vi "frontend2.vi"() -> ()   [LabVIEW 2011]
uses:
  custom_modules/typedefs/preset_control_cluster.ctl
  custom_modules/typedefs/control_cluster.ctl
  custom_modules/typedefs/origin_controls.ctl
  custom_modules/typedefs/single_step_controls.ctl
  custom_modules/typedefs/camera_settings_new.ctl
  custom_modules/typedefs/states_v2.ctl
  <vilib>/event_ctls.llb/eventvkey.ctl
  custom_modules/typedefs/dynamic_data.ctl
  <vilib>/vision/Image Controls.llb/IMAQ Image.ctl
  custom_modules/typedefs/image_type.ctl
  <vilib>/Utility/error.llb/DialogType.ctl
  stage_modules/Globals.vi
  <userlib>/qcam/QCam.llb/QCam Grab Abort.vi
  <vilib>/vision/NI_Vision_Development_Module.lvlib
panel:
  in  "test start time":u32
  out "abort test":bool
  out "error display":errorcluster
  in  "Tab Control":enum32{"Settings", "Advanced"}(tab)
  in  "Preset controls":T1 {"Presets" items=["500sep.preset", "test1.preset", "test2.preset", "test3.preset"]}
  in  "Movement controls":T2={"Nx"=10, "Ny"=10, "X separation"=100, "Y separation"=100}
  in  "File name base":string="<title>_<length>_<sampleID>_<stain>"
  in  "Run test button":bool
  in  "close button":bool
  in  "Origin controls":T3
  in  "Single step controls":T4
  in  "Camera settings":T5={"Gain"=1.0, "Exposure (s)"=0.05, "Preview binning"=2, "Capture binning"=0, "auto expose button"=FALSE} {"Capture binning" items=["1x1", "2x2", "4x4", "8x8"]; "Preview binning" items=["1x1", "2x2", "4x4", "8x8"]; "Exposure (s)" scale=1e-05..1000.0 scale format="%^#_1e"; "Gain" scale=0.451..21.5 scale format="%#_3g"}
  out "Histogram":T6(graph)
  out "Preview":T7(plugin-control)
  in  "camera button":bool
  in  "Image Output directory":path=path "C:/Users/0800706m/Documents/output"
  out "connection indicator":bool
  out "Scan map viewer":T7(plugin-control)
  out "elapsed time":string
  out "estimated remaining":string
  in  "Well numbering mode":u16(ring)=1 items=["X and Y numbers", "Numbers and letters"]
  in  "No. of wells Y":i32=1
  in  "No. of wells X":i32=1
  in  "Well separation Y":dbl=899.0
  in  "Well separation X":dbl=899.0
  in  "PC connection port":u16(ring)=3 items=["PCI board", "COM 1", "TPL1", "COM3"]
  in  "No. of images in focal stack":i32=1
  in  "Focal stack separation":dbl=1.0
  in  "Preset directory":path=path "C:/Users/0800706m/Documents/microscope_software/presets"
  in  "Additional delay between captures (ms)":dbl=1000.0
  in  "emergency stop":bool
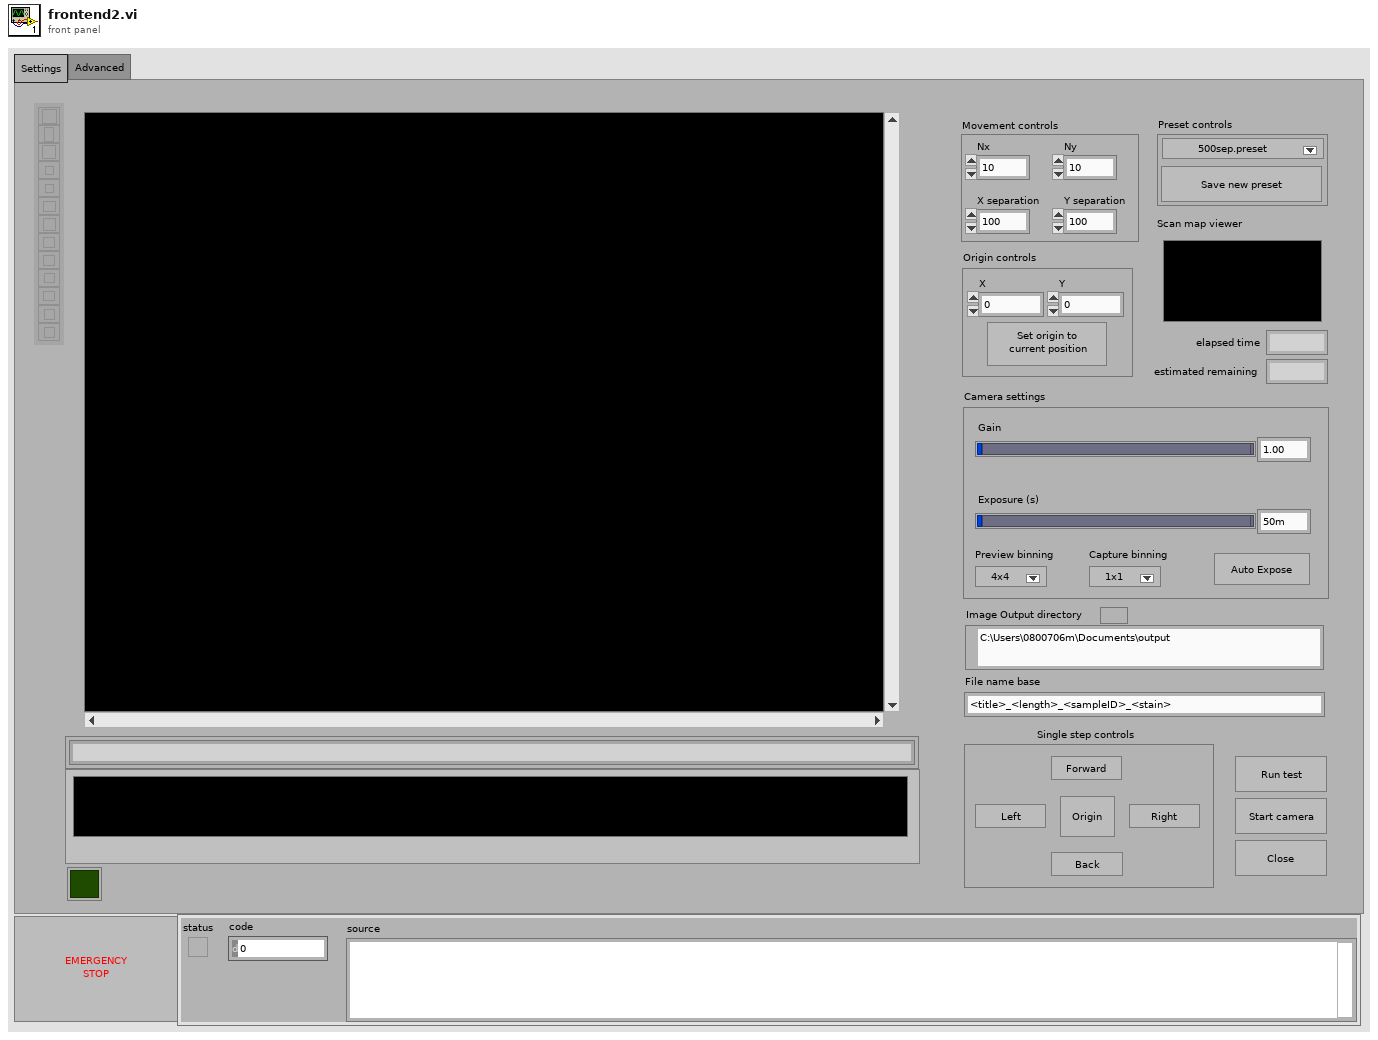
[diagram p1: front panel]
types:
  T1 = typedef "preset_control_cluster.ctl" = cluster{"Presets":u16, "save preset button":bool}
  T2 = typedef "control_cluster.ctl" = cluster{"Nx":i32, "Ny":i32, "X separation":i32, "Y separation":i32}
  T3 = typedef "origin_controls.ctl" = cluster{"X":dbl, "Y":dbl, "set origin button":bool}
  T4 = typedef "single_step_controls.ctl" = cluster{"move to origin button":bool, "Left":bool, "Right":bool, "Back":bool, "Forward":bool}
  T5 = typedef "camera_settings_new.ctl" = cluster{"Gain":dbl, "Exposure (s)":dbl, "Preview binning":u16, "Capture binning":u16, "auto expose button":bool}
  T6 = cluster{"Starting Value":sgl, "Incremental Value":sgl, "Histogram":u32[]}
  T7 = typedef "IMAQ Image.ctl" = refnum<image>
  T8 = typedef "states_v2.ctl" = enum16{"Init", "Preview", "Test init", "Test run", "Test clean", "Close"}
  T9 = typedef "dynamic_data.ctl" = cluster{"PRIORLib.IScanOut":refnum<k7>, "PRIORLib.IStageOut":refnum<k7>, "PRIORLib.IFilterOut":refnum<k7>, "PRIORLib.IZOut":refnum<k7>, "cameraID":u32, "Image Out":T7, "focal map fileref":refnum<file>, "Scan map":T7, "start time":u32}
  T10 = enum8{"Enabled", "Disabled", "Disabled and Grayed Out"}
  T11 = typedef "image_type.ctl" = enum16{"preview_image", "capture_image"}
  T12 = enum32{"gain", "offset", "exposure", "binning", "horizontal binning", "vertical binning", "readout speed", "trigger type", "lcd filter", "cooler", "exposure red", "exposure blue", "image format", "roi x", "roi y", "roi width", "roi height", "reserved1", "shutter state", "reserved2", "sync-b out", "reserved3", "intensifier gain", "trigger delay", "camera mode", "normalized gain", "normalized intenifier gain DB", "doPostProcessing", "postProcessGainRed", "postProcessGainGreen", "postProcessGainBlue", "postProcessBayerAlgorithm", "postProcessImageFormat", "fan", "blackout mode", "high sensitivity", "Readout Port", "EM Gain", "open delay", "close delay", "clearing mode"}
  T13 = enum16{"open", "replace", "create", "open or create", "replace or create", "replace or create with confirmation"}
  T14 = typedef "Image Type" = u32
  T15 = cluster{"Value":bool, "Value":bool, "Value":bool, "Value":bool, "Value":bool}
  T16 = cluster{"Global Rectangle":i32[], "Contours":cluster{"Contour Type":u32, "ROI Type":u32, "Points":i32[]}[]}
  T17 = typedef "DialogType.ctl" = u16
  T18 = cluster{"stage adjusted":bool, "stage adjusted":bool, "stage adjusted":bool, "stage adjusted":bool, "stage adjusted":bool}
  T19 = cluster{"Focus position":dbl, "Number of captures":i32}
  T20 = typedef "eventvkey.ctl" = enum16{"ASCII", "Enter", "Return", "Shift", "Ctrl", "Alt", "Cmd", "Opt", "Caps", "NumLock", "Clear", "Break", "Up", "Down", "Left", "Right", "Insert", "Delete", "Home", "End", "PageUp", "PageDown", "Escape", "Help", "Pause", "ScrollLock", "F1", "F2", "F3", "F4", "F5", "F6", "F7", "F8", "F9", "F10", "F11", "F12", "F13", "F14", "F15", "F16", "F17", "F18", "F19", "F20", "F21", "F22", "F23", "F24", "Play", "VolumeUp", "VolumeDown", "Mute", "Two Byte Char"}
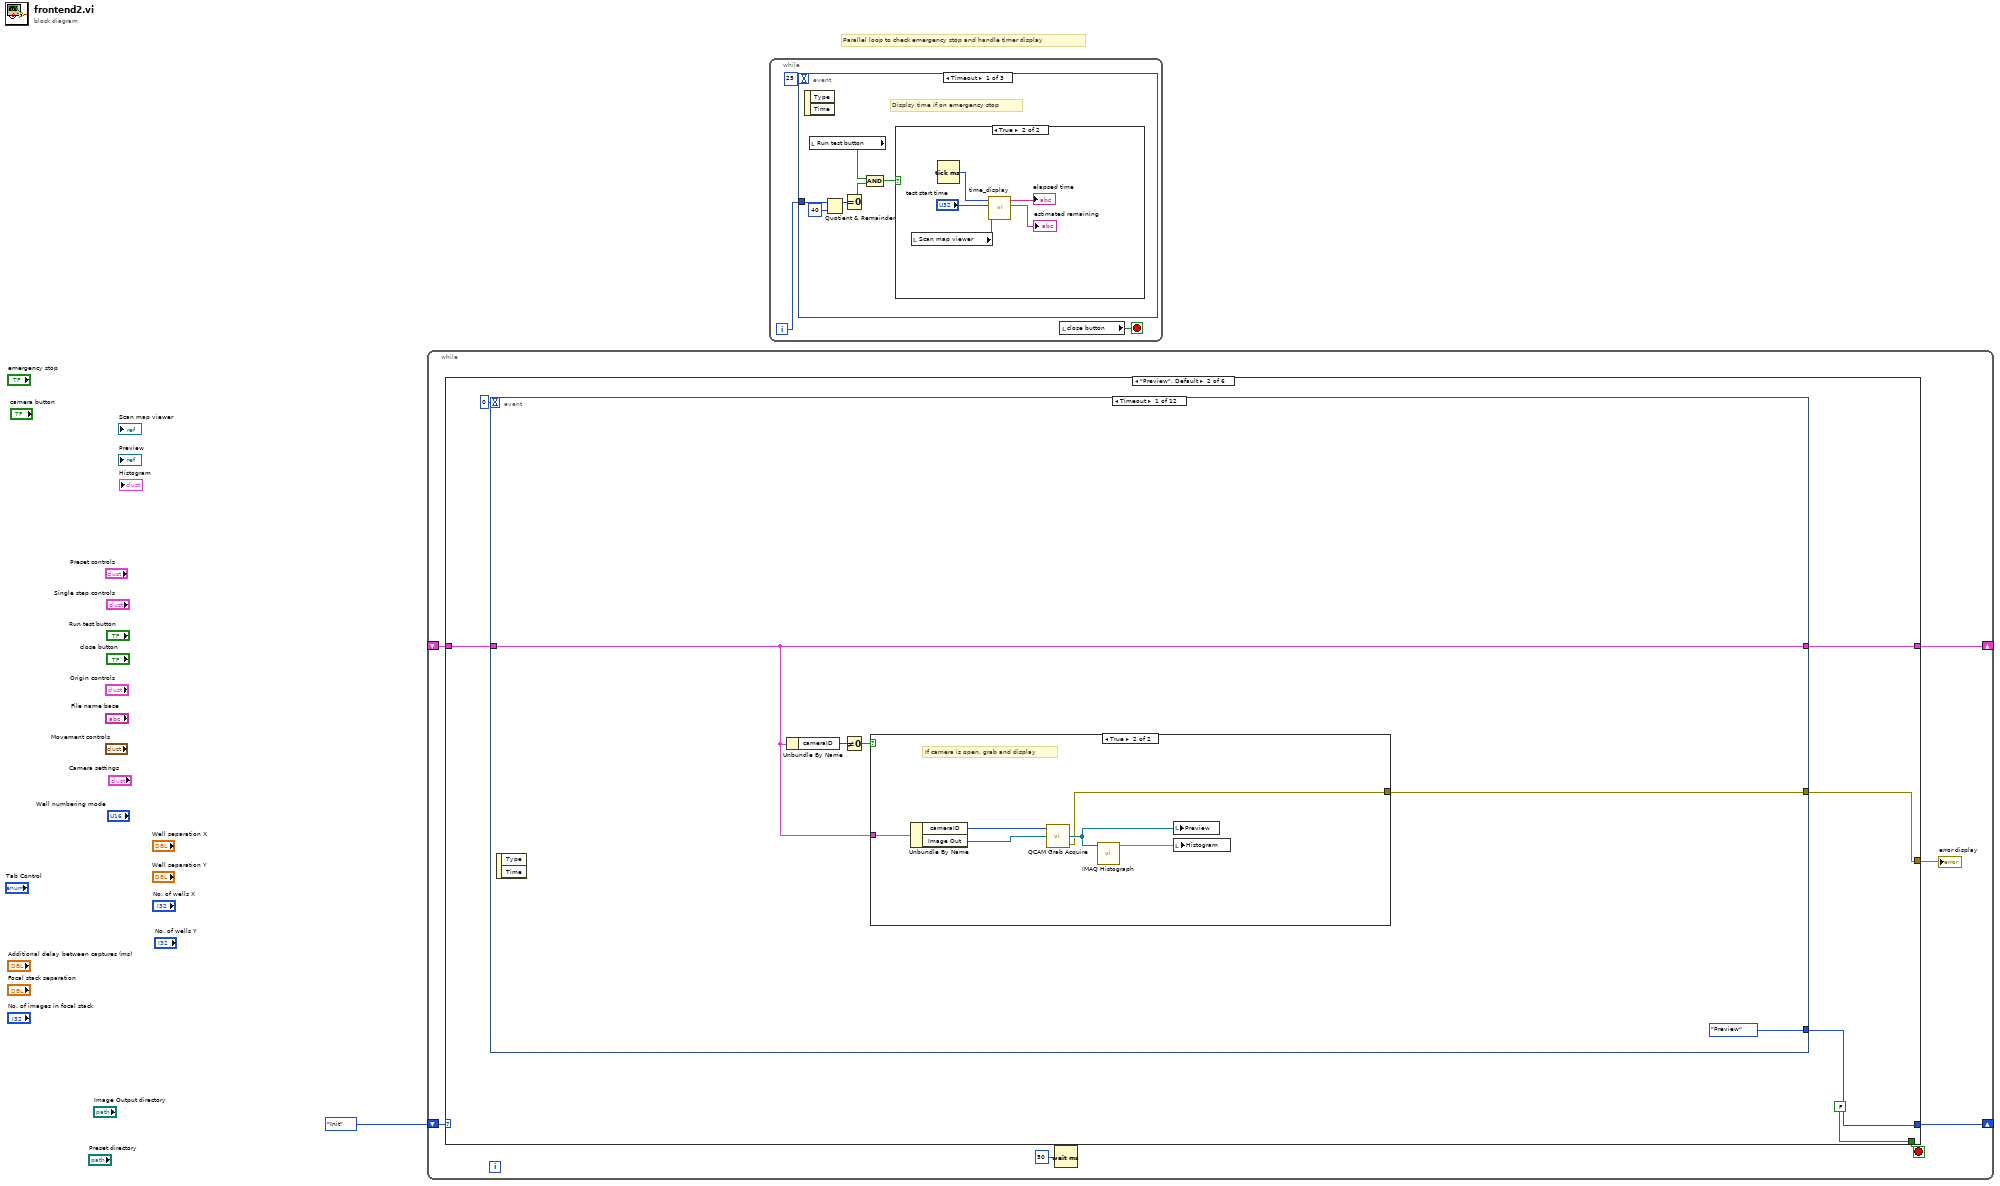
[diagram p0: block diagram]
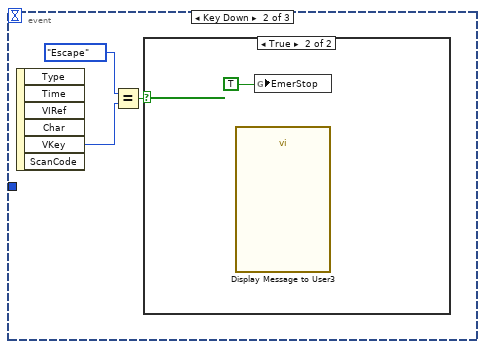
[diagram p3: hidden frame]
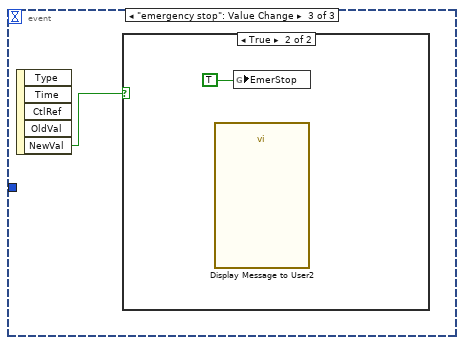
[diagram p5: hidden frame]
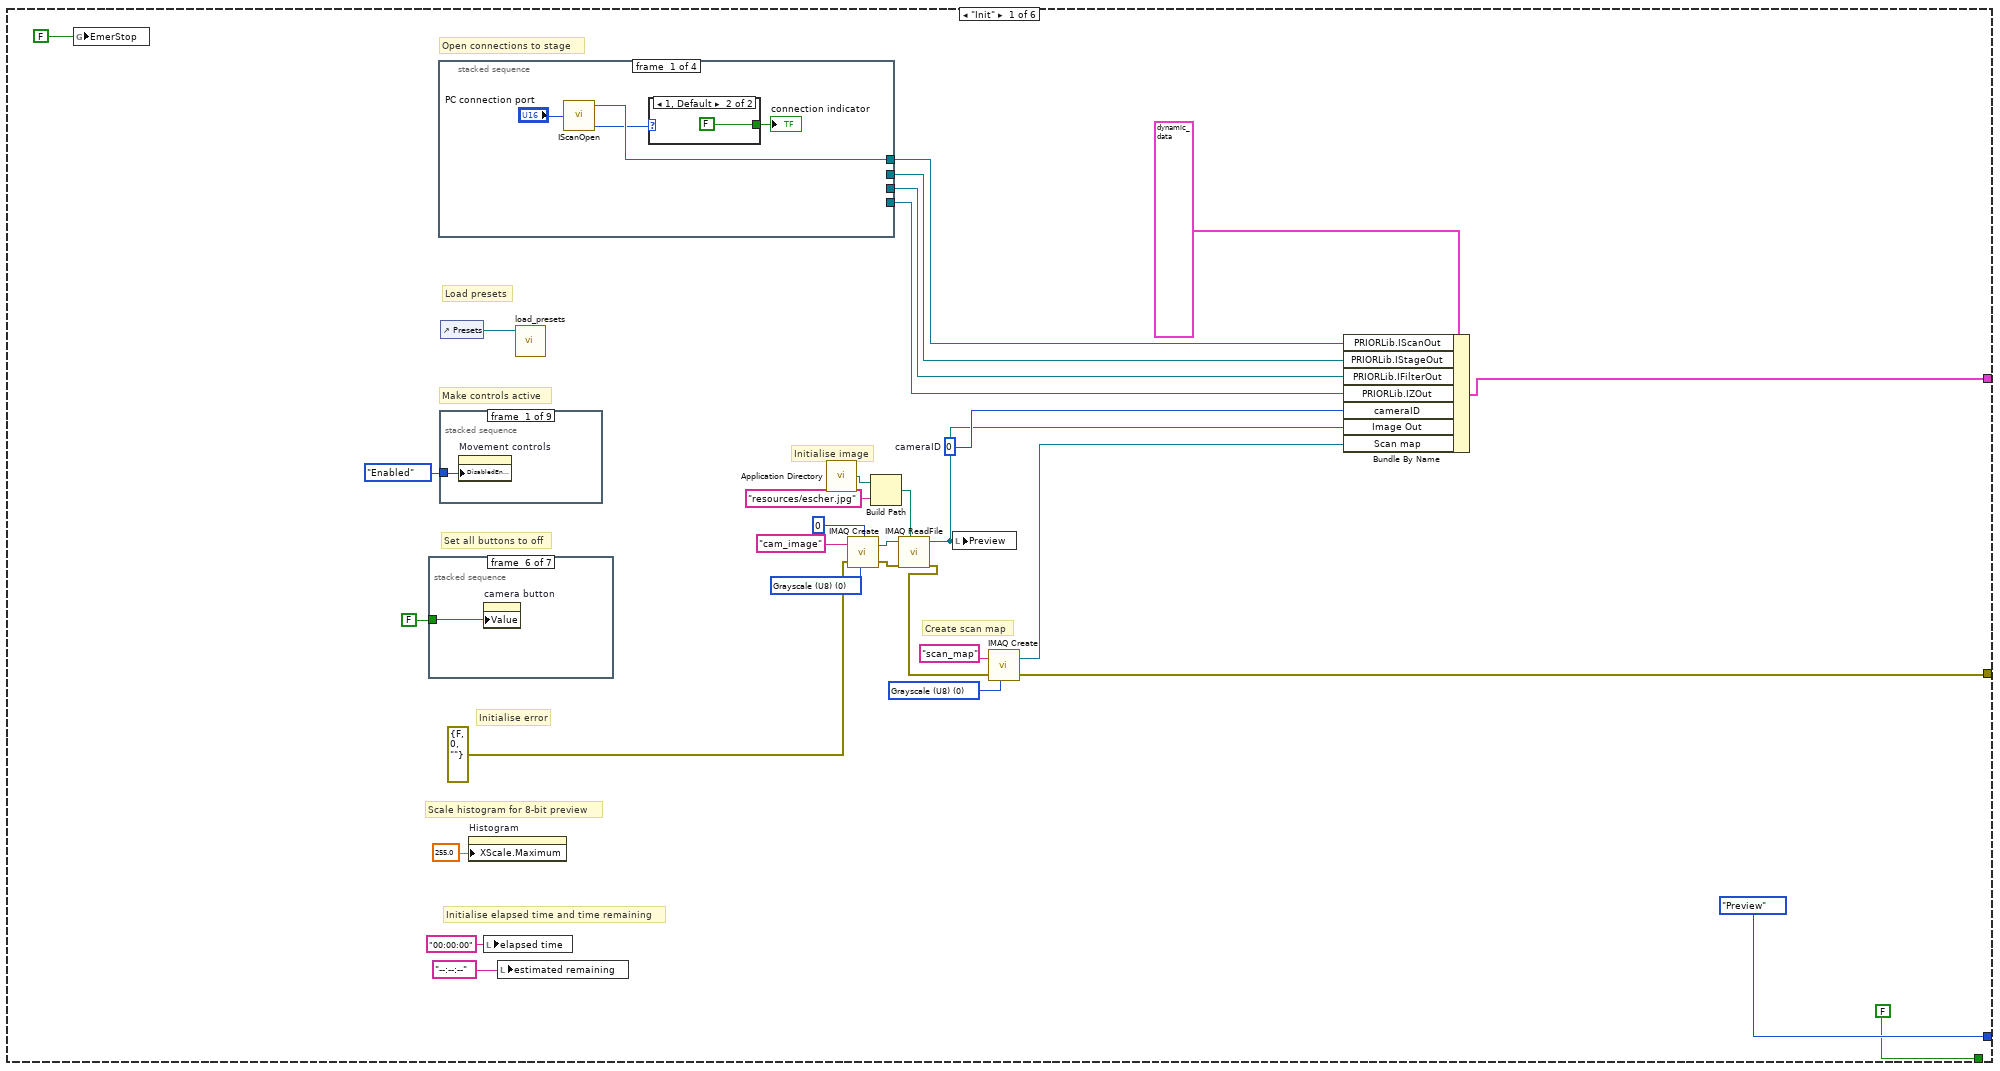
[diagram p7: hidden frame]
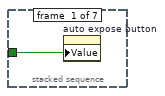
[diagram p8: hidden frame]
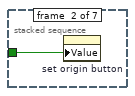
[diagram p9: hidden frame]
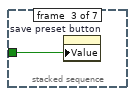
[diagram p10: hidden frame]
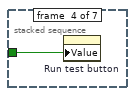
[diagram p11: hidden frame]
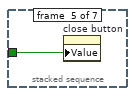
[diagram p12: hidden frame]
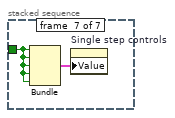
[diagram p13: hidden frame]
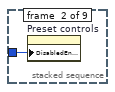
[diagram p14: hidden frame]
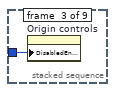
[diagram p15: hidden frame]
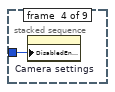
[diagram p16: hidden frame]
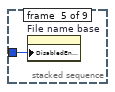
[diagram p17: hidden frame]
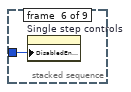
[diagram p18: hidden frame]
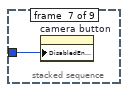
[diagram p19: hidden frame]
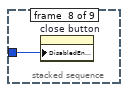
[diagram p20: hidden frame]
diagram:
  # "Parallel loop to check emergency stop and handle timer display"
  n1 = while {
    shift-right: [w7] -> _
    shift-left: states_v2."Init" -> [w8]
    shift-right: [w5] -> _
    shift-left: _ -> [w2]
    stop <- w6 stop-if-true
    n2 = case shown="\"Preview\", Default" w8 {
      tunnel: [states_v2."Preview" w72 w315 states_v2."Test clean" states_v2."Preview" states_v2."Close"] -> w7
      tunnel: [FALSE FALSE FALSE FALSE FALSE TRUE] -> w6
      tunnel: [w19 w70 w280 w341 w542 T9 {"PRIORLib.IScanOut"=refnum, "PRIORLib.IStageOut"=refnum, "PRIORLib.IFilterOut"=refnum, "PRIORLib.IZOut"=refnum, "cameraID"=0, "Image Out"=refnum, "focal map fileref"=refnum, "Scan map"=refnum, "start time"=0}] -> w5
      tunnel: w2 -> [_ w69 w281 w341 w534 w558]
      tunnel: [w13 w68 w279 _ w531 w556] -> w3
      frame "Init" {
        w17 = T14 0 items=["Grayscale (U8)", "Grayscale (I16)", "Grayscale (SGL)", "Complex (CSG)", "RGB (U32)", "HSL (U32)", "RGB (U64)", "Grayscale (U16)"] ("Image Type")
        w29 = T14 0 items=["Grayscale (U8)", "Grayscale (I16)", "Grayscale (SGL)", "Complex (CSG)", "RGB (U32)", "HSL (U32)", "RGB (U64)", "Grayscale (U16)"] ("Image Type")
        w28 = u32 0  # cameraID
        # "Initialise elapsed time and time remaining"
        # "Create scan map"
        # "Initialise image"
        # "Scale histogram for 8-bit preview"
        # "Initialise error"
        # "Set all buttons to off"
        # "Make controls active"
        # "Open connections to stage"
        # "Load presets"
        n3 = global write "Globals.vi" "EmerStop"(FALSE) -> ()
        n4 = stacked-sequence {
          tunnel: FALSE ("Value") -> [w40 w41 w42 w43 w44 w45 w46]
          frame #0 {
            n5 = property on="auto expose button" class="Bool (strict)"("Value"=w40) -> ()  [unwired: 2 in, 2 out]
          }
          frame #1 {
            n6 = property on="set origin button" class="Bool (strict)"("Value"=w41) -> ()  [unwired: 2 in, 2 out]
          }
          frame #2 {
            n7 = property on="save preset button" class="Bool (strict)"("Value"=w42) -> ()  [unwired: 2 in, 2 out]
          }
          frame #3 {
            n8 = property on="Run test button" class="Bool (strict)"("Value"=w43) -> ()  [unwired: 2 in, 2 out]
          }
          frame #4 {
            n9 = property on="close button" class="Bool (strict)"("Value"=w44) -> ()  [unwired: 2 in, 2 out]
          }
          frame #5 {
            n10 = property on="camera button" class="Bool (strict)"("Value"=w45) -> ()  [unwired: 2 in, 2 out]
          }
          frame #6 {
            n11 = Bundle("Value"=w46, "Value"=w46, "Value"=w46, "Value"=w46, "Value"=w46) -> (w47:T15)  [unwired: 1 in]
            n12 = property on="Single step controls" class="Clust (strict)"("Value"=w47) -> ()  [unwired: 2 in, 2 out]
          }
        }
        n13 = stacked-sequence {
          tunnel: [w60 _ _ _] -> w10
          tunnel: [_ w63 _ _] -> w35
          tunnel: [_ _ w64 _] -> w34
          tunnel: [_ _ _ w65] -> w33
          frame #0 {
            n14 = call "IScanOpen.vi"("Port"="PC connection port") -> ("PRIORLib.IScanOut"=w60:refnum<k7>, "Return"=w59:i32)  [unwired: 1 out]
            n15 = case shown="1, Default" w59 {
              tunnel: [TRUE ("connection indicator") FALSE ("connection indicator")] -> w57
              frame 0 {
              }
              frame 1, Default {
              }
            }
            "connection indicator" <- w57
          }
          frame #1 {
            n16 = call "IStageOpen.vi"() -> ("PRIORLib.IStageOut"=w63:refnum<k7>)  [unwired: 1 in, 1 out]
          }
          frame #2 {
            n17 = call "IFilterOpen.vi"() -> ("PRIORLib.IFilterOut"=w64:refnum<k7>)  [unwired: 1 in, 1 out]
          }
          frame #3 {
            n18 = call "IZOpen.vi"() -> ("PRIORLib.IZOut"=w67:refnum<k7>)  [unwired: 1 in, 1 out]
            n19 = call "IZMaxSpeed.vi"("ZSpeed"=50.0, "PRIORLib.IZIn"=w67) -> ("PRIORLib.IZOut"=w65:refnum<k7>)  [unwired: 1 out]
          }
        }
        n20 = stacked-sequence {
          tunnel: T10."Enabled" ("Disabled") -> [w48 w49 w50 w51 w52 w53 w54 w55 w56]
          frame #0 {
            n21 = property on="Movement controls" class="Clust (strict)"("DisabledEnum"=w48) -> ()  [unwired: 2 in, 2 out]
          }
          frame #1 {
            n22 = property on="Preset controls" class="Clust (strict)"("DisabledEnum"=w49) -> ()  [unwired: 2 in, 2 out]
          }
          frame #2 {
            n23 = property on="Origin controls" class="Clust (strict)"("DisabledEnum"=w50) -> ()  [unwired: 2 in, 2 out]
          }
          frame #3 {
            n24 = property on="Camera settings" class="Clust (strict)"("DisabledEnum"=w51) -> ()  [unwired: 2 in, 2 out]
          }
          frame #4 {
            n25 = property on="File name base" class="Str"("DisabledEnum"=w52) -> ()  [unwired: 2 in, 2 out]
          }
          frame #5 {
            n26 = property on="Single step controls" class="Clust (strict)"("DisabledEnum"=w53) -> ()  [unwired: 2 in, 2 out]
          }
          frame #6 {
            n27 = property on="camera button" class="Bool (strict)"("DisabledEnum"=w54) -> ()  [unwired: 2 in, 2 out]
          }
          frame #7 {
            n28 = property on="close button" class="Bool (strict)"("DisabledEnum"=w55) -> ()  [unwired: 2 in, 2 out]
          }
          frame #8 {
            n29 = property on="Image Output directory" class="Path"("DisabledEnum"=w56) -> ()  [unwired: 2 in, 2 out]
          }
        }
        n30 = control-ref of="Presets"() -> (w37:refnum<vi>)
        n31 = property on="Histogram" class="WFGraph (strict)"("XScale.Maximum"=255.0 ("X Scale.Range:Maximum")) -> ()  [unwired: 2 in, 2 out]
        n32 = local write "elapsed time"("00:00:00" ("date/time string")) -> ()
        n33 = local write "estimated remaining"("--:--:--" ("estimated time remaining")) -> ()
        n34 = call "load_presets.vi"("Ring in"=w37) -> ()  [unwired: 11 in]
        n35 = call <vilib>:"Application Directory.vi"() -> ("Application Directory"=w23:path)
        n36 = call "IMAQ Create"("Border Size"=0, "Image Name"="cam_image", "Image Type"=w29, "error in (no error)"=errorcluster {"status"=FALSE, "code"=0, "source"=""} ("error display")) -> ("New Image"=w26:T7, "error out"=w25:errorcluster)  [unwired: 1 in]
        n37 = Build Path(base path=w23, name or relative path="resources/escher.jpg") -> (appended path=w21:path)
        n38 = call "IMAQ ReadFile"("File Path"=w21, "error in (no error)"=w25, "Image"=w26) -> ("error out"=w14:errorcluster, "Image Out"=w24:T7)  [unwired: 4 in, 3 out]
        n39 = local write "Preview"(w24) -> ()
        n40 = call "IMAQ Create"("Image Name"="scan_map", "Image Type"=w17, "error in (no error)"=w14) -> ("New Image"=w16:T7, "error out"=w13:errorcluster)  [unwired: 2 in]
        n41 = Bundle By Name(cluster=T9 {"PRIORLib.IScanOut"=refnum, "PRIORLib.IStageOut"=refnum, "PRIORLib.IFilterOut"=refnum, "PRIORLib.IZOut"=refnum, "cameraID"=0, "Image Out"=refnum, "focal map fileref"=refnum, "Scan map"=refnum, "start time"=0} ("output cluster"), "PRIORLib.IScanOut"=w10, "PRIORLib.IStageOut"=w35, "PRIORLib.IFilterOut"=w34, "PRIORLib.IZOut"=w33, "cameraID"=w28, "Image Out"=w24, "Scan map"=w16) -> (w19:T9)
      }
      frame "Preview", Default {
        n42 = event shown="[0] Timeout" {
          selector: _ -> [_ _ _ _ _ _ _ _ _ _ _ _]
          dyn-events: _ -> [_ _ _ _ _ _ _ _ _ _ _ _]
          timeout: 0 -> [_ _ _ _ _ _ _ _ _ _ _ _]
          tunnel: [states_v2."Preview" states_v2."Close" states_v2."Preview" states_v2."Preview" states_v2."Preview" states_v2."Preview" states_v2."Preview" w194 states_v2."Preview" states_v2."Preview" states_v2."Preview" states_v2."Preview"] -> w72
          tunnel: w69 -> [w75 w85 w90 w114 w132 w142 w165 w195 w199 w206 w215 w227]
          tunnel: [w75 w85 w88 w114 w132 w145 w165 w195 w199 w206 w215 w227] -> w70
          tunnel: [w74 _ w87 w113 w128 w140 w160 _ _ _ w213 _] -> w68
          event Timeout {
            n43 = event-data() -> ()  [unwired: 1 in, 2 out]
            n44 = Unbundle By Name(w75) -> ("cameraID"=w76:u32)
            n45 = Not Equal To 0?(x=w76) -> (x != 0?=w77:bool)
            n46 = case shown="True" w77 {
              tunnel: w75 -> [_ w82]
              tunnel: [_ w79] -> w74
              frame False {
              }
              frame True {
                # "If camera is open, grab and display"
                n47 = Unbundle By Name(w82) -> ("cameraID"=w84:u32, "Image Out"=w83:T7)
                n48 = call <userlib>:"QCAM Grab Acquire.vi"("Image"=w83, "cameraId"=w84) -> ("error out"=w79:errorcluster, "Image Out"=w81:T7)  [unwired: 1 in, 1 out]
                n49 = call "IMAQ Histograph"("Image"=w81) -> ("Histogram Graph"=w80:T6)  [unwired: 7 in, 3 out]
                n50 = local write "Preview"(w81) -> ()
                n51 = local write "Histogram"(w80) -> ()
              }
            }
          }
          event "close button": Value Change {
            n52 = event-data() -> ()  [unwired: 1 in, 5 out]
          }
          event "camera button": Value Change {
            n53 = event-data() -> ("NewVal"=w91:bool)  [unwired: 1 in, 4 out]
            n54 = case shown="True" w91 {
              tunnel: w90 -> [w94 w105]
              tunnel: [w93 w112] -> w88
              tunnel: [w92 w104] -> w87
              frame False {
                # "Close camera if button unclicked"
                n55 = stacked-sequence {
                  tunnel: w94 -> [_ w97 w103]
                  tunnel: [_ _ w102] -> w93
                  tunnel: [_ w96 _] -> w92
                  frame #0 {
                    # "BAD!!! Get rid of this !"
                    n56 = global write "QCam Grab Abort.vi" "Grab Abort"(TRUE ("Grab Abort")) -> ()
                  }
                  frame #1 {
                    # "Stop capture and camera"
                    n57 = Unbundle By Name(w97) -> ("cameraID"=w98:u32)
                    n58 = call <userlib>:"QCAM Grab Stop.vi"("cameraId"=w98) -> ("error out"=w99:errorcluster, "cameraId Out"=w100:u32)  [unwired: 1 in]
                    n59 = call <userlib>:"QCAM Close.vi"("error in (no error)"=w99, "cameraId"=w100) -> ("error out"=w96:errorcluster)  [unwired: 1 in]
                  }
                  frame #2 {
                    # "set camera ID to 0"
                    n60 = Bundle By Name(cluster=w103, "cameraID"=u32 0) -> (w102:T9)
                  }
                }
              }
              frame True {
                # "Free original image"
                # "Start camera"
                # "Open camera if button clicked"
                n61 = Unbundle By Name(w105) -> ("Image Out"=w107:T7)
                n62 = call "IMAQ Dispose"("Image"=w107) -> ("error out"=w106:errorcluster)  [unwired: 5 in]
                n63 = local read "Camera settings"() -> (w108:T5)
                n64 = call "start_camera_new.vi"("error in (no error)"=w106, "image type"=image_type."preview_image", "Camera settings"=w108) -> ("error out"=w104:errorcluster, "cameraId out"=w110:u32, "Refnum out"=w109:T7)  [unwired: 5 in, 1 out]
                n65 = Bundle By Name(cluster=w105, "cameraID"=w110, "Image Out"=w109) -> (w112:T9)
              }
            }
          }
          event Value Change {
            # "Handle gain changes"
            n66 = event-data() -> ("NewVal"=w116:dbl)  [unwired: 1 in, 4 out]
            n67 = Unbundle By Name(w114) -> ("cameraID"=w115:u32)
            n68 = Not Equal To 0?(x=w115) -> (x != 0?=w118:bool)
            n69 = case shown="False" w118 {
              tunnel: w116 -> [_ w121]
              tunnel: w115 -> [_ w120]
              tunnel: [_ w119] -> w113
              frame False {
              }
              frame True {
                n70 = Divide(x=w121, y=0.451) -> (x/y=w125:dbl)
                n71 = Logarithm Base X(1:1.000944118 ("x"), 2:w125) -> (0:w123:dbl)
                n72 = To Long Integer(number=w123) -> (32bit integer=w122:i32)
                n73 = call <userlib>:"QCAM SetParam.vi"("value"=w122, "parameter key"=T12."gain", "cameraId"=w120) -> ("error out"=w119:errorcluster)  [unwired: 1 in, 1 out]
              }
            }
          }
          event Value Change {
            # "Handle exposure changes"
            n74 = event-data() -> ("NewVal"=w130:dbl)  [unwired: 1 in, 4 out]
            n75 = Unbundle By Name(w132) -> ("cameraID"=w129:u32)
            n76 = Not Equal To 0?(x=w129) -> (x != 0?=w133:bool)
            n77 = case shown="True" w133 {
              tunnel: w130 -> [_ w136]
              tunnel: w129 -> [_ w135]
              tunnel: [_ w134] -> w128
              frame False {
              }
              frame True {
                n78 = Multiply(x=w136, y=1000000.0 ("x")) -> (x*y=w139:dbl)
                n79 = call <userlib>:"QCAM SetParam.vi"("value"=w139, "parameter key"=T12."exposure", "cameraId"=w135) -> ("error out"=w134:errorcluster)  [unwired: 1 in, 1 out]
              }
            }
          }
          event Value Change {
            # "Handle binning changes"
            n80 = event-data() -> ()  [unwired: 1 in, 5 out]
            n81 = Unbundle By Name(w142) -> ("cameraID"=w144:u32)
            n82 = Not Equal To 0?(x=w144) -> (x != 0?=w143:bool)
            n83 = case shown="True" w143 {
              tunnel: w142 -> [w146 w147]
              tunnel: [w146 w159] -> w145
              tunnel: [_ w158] -> w140
              frame False {
              }
              frame True {
                # "start camera with new binning"
                # "stop camera and free image"
                n84 = Unbundle By Name(w147) -> ("cameraID"=w155:u32, "Image Out"=w156:T7)
                n85 = call <userlib>:"QCAM Grab Stop.vi"("cameraId"=w155) -> ("error out"=w154:errorcluster, "cameraId Out"=w153:u32)  [unwired: 1 in]
                n86 = call <userlib>:"QCAM Close.vi"("error in (no error)"=w154, "cameraId"=w153) -> ("error out"=w157:errorcluster)  [unwired: 1 in]
                n87 = call "IMAQ Dispose"("Image"=w156, "error in (no error)"=w157) -> ("error out"=w148:errorcluster)  [unwired: 4 in]
                n88 = local read "Camera settings"() -> (w149:T5)
                n89 = call "start_camera_new.vi"("error in (no error)"=w148, "image type"=image_type."preview_image", "Camera settings"=w149) -> ("error out"=w158:errorcluster, "cameraId out"=w151:u32, "Refnum out"=w150:T7)  [unwired: 5 in, 1 out]
                n90 = Bundle By Name(cluster=w147, "cameraID"=w151, "Image Out"=w150) -> (w159:T9)
              }
            }
          }
          event Value Change {
            # "Auto expose from ROI or full image if there is no ROI"
            # "Update exposure slider"
            n91 = event-data() -> ()  [unwired: 1 in, 5 out]
            n92 = Unbundle By Name(w165) -> ("cameraID"=w168:u32, "Image Out"=w167:T7)
            n93 = property on="Preview" class="ImageControl"() -> ("ROI"=w169:T16)  [unwired: 2 in, 2 out]
            n94 = Unbundle(w169) -> ("Global Rectangle"=w172:i32[])  [unwired: 1 out]
            n95 = Array Size(array=w172) -> (size(s)=w173:i32)
            n96 = Not Equal To 0?(x=w173) -> (x != 0?=w174:bool)
            n97 = case shown="True" w174 {
              tunnel: w172 -> [_ w190]
              tunnel: [w182 w189] -> w175
              tunnel: [w182 w188] -> w176
              tunnel: [w183 w187] -> w177
              tunnel: [w184 w186] -> w178
              tunnel: w167 -> [w181 _]
              tunnel: [w180 errorcluster {"status"=FALSE, "code"=0, "source"=""} ("error out")] -> w164
              frame False {
                w182 = 0
                n98 = call "IMAQ GetImageSize"("Image"=w181) -> ("Y Resolution"=w184:i32, "X Resolution"=w183:i32, "error out"=w180:errorcluster)  [unwired: 3 in]
              }
              frame True {
                n99 = Index Array(array=w190) -> (element #1=w189:i32, element #2=w188:i32, element #3=w192:i32, element #4=w191:i32)  [unwired: 4 in]
                n100 = Subtract(x=w192, y=w189) -> (x-y=w187:i32)
                n101 = Subtract(x=w191, y=w188) -> (x-y=w186:i32)
              }
            }
            n102 = call <userlib>:"QCAM AutoExpose.vi"("xOrig"=w175, "cameraId"=w168, "yOrig"=w176, "width"=w177, "error in (no error)"=w164, "height"=w178) -> ("cameraId out"=w171:u32, "error out"=w170:errorcluster)  [unwired: 1 in]
            n103 = call <userlib>:"QCAM GetParam.vi"("cameraId in"=w171, "parameter key"=T12."exposure", "error in (no error)"=w170) -> ("value out"=w161:u32, "error out"=w160:errorcluster)  [unwired: 3 out]
            n104 = Divide(x=w161, y=u32 1000000 ("x")) -> (x/y=w163:dbl)
            n105 = property on="Exposure (s)" class="Slide (strict)"("Value"=w163) -> ()  [unwired: 2 in, 2 out]
          }
          event "Run test button": Value Change {
            # "Go to test mode"
            n106 = event-data() -> ("NewVal"=w193:bool)  [unwired: 1 in, 4 out]
            n107 = case shown="True" w193 {
              tunnel: [states_v2."Preview" states_v2."Test init"] -> w194
              frame False {
              }
              frame True {
              }
            }
          }
          event Value Change {
            # "Get current position from stage and use as origin"
            n108 = event-data() -> ()  [unwired: 1 in, 5 out]
            n109 = Unbundle By Name(w199) -> ("PRIORLib.IStageOut"=w200:refnum<k7>)
            n110 = stacked-sequence {
              tunnel: w200 -> [w203 _]
              frame #0 {
                # "Change origin if button has been pressed"
                n111 = invoke class="IStage" method="GetPosition"(reference=w203) -> ("XPos"=w201:dbl, "YPos"=w202:dbl)  [unwired: 4 in, 3 out]
                n112 = property on="X" class="DigNum (strict)"("Value"=w201) -> ()  [unwired: 2 in, 2 out]
                n113 = property on="Y" class="DigNum (strict)"("Value"=w202) -> ()  [unwired: 2 in, 2 out]
              }
              frame #1 {
                # "Restore button"
                n114 = property on="set origin button" class="Bool (strict)"("Value"=FALSE ("set origin button")) -> ()  [unwired: 2 in, 2 out]
              }
            }
          }
          event Value Change {
            # "Save current settings as preset"
            n115 = event-data() -> ()  [unwired: 1 in, 5 out]
            n116 = stacked-sequence {
              frame #0 {
                w208 = T17 0 items=["no dialog", "OK message", "continue or stop message", "OK message + warnings", "continue/stop + warnings"] ("type of dialog (OK msg:1)")
                # "Save controls as XML preset and ignore errors"
                n117 = local read "Movement controls"() -> (w207:T2)
                n118 = Flatten To XML(anything=w207) -> (xml string=w210:string)
                n119 = Write to Text File(text=w210) -> (error out=w209:errorcluster)  [unwired: 3 in, 2 out]
                n120 = call <vilib>:"Simple Error Handler.vi"("type of dialog (OK msg:1)"=w208, "error in (no error)"=w209) -> ()  [unwired: 3 in, 5 out]
              }
              frame #1 {
                # "Reload preset list"
                n121 = control-ref of="Presets"() -> (w211:refnum<vi>)
                n122 = call "load_presets.vi"("Ring in"=w211) -> ()  [unwired: 11 in]
              }
              frame #2 {
                # "Restore button"
                n123 = property on="save preset button" class="Bool (strict)"("Value"=FALSE) -> ()  [unwired: 2 in, 2 out]
              }
            }
          }
          event Value Change {
            # "Get currently selected preset and load into controls"
            # "List \".preset\" files in preset folder"
            n124 = event-data() -> ("NewVal"=w216:u16)  [unwired: 1 in, 4 out]
            n125 = local read "Preset directory"() -> (w225:path)
            n126 = List Folder(path=w225, pattern="*.preset") -> (filenames=w219:string[])  [unwired: 2 in, 3 out]
            n127 = Index Array(array=w219, index=w216) -> (element=w218:string)
            n128 = Build Path(base path=w225, name or relative path=w218) -> (appended path=w222:path)
            n129 = Read from Text File(file (use dialog)=w222) -> (text=w224:string, error out=w223:errorcluster)  [unwired: 3 in, 2 out]
            n130 = Unflatten From XML(xml string=w224, type=T2 {"Nx"=0, "Ny"=0, "X separation"=0, "Y separation"=0} ("controls"), error in (no error)=w223) -> (value=w217:T2, error out=w213:errorcluster)
            n131 = local write "Movement controls"(w217) -> ()
          }
          event Value Change {
            # "Cycle through buttons and execute the one that has been pressed"
            # "Move stage by 1 step.\nSize of step is determined by movement controls"
            n132 = event-data() -> ()  [unwired: 1 in, 5 out]
            n133 = Unbundle By Name(w227) -> ("PRIORLib.IScanOut"=w226:refnum<k7>)
            n134 = local read "Movement controls"() -> (w231:T2)
            n135 = local read "Single step controls"() -> (w228:T4)
            n136 = Unbundle By Name(w231) -> ("X separation"=w229:i32, "Y separation"=w230:i32)
            n137 = stacked-sequence {
              tunnel: w226 -> [w235 w241 w249 w256 w264 _]
              tunnel: w228 -> [w233 w244 w252 w259 w267 _]
              tunnel: w230 -> [_ _ _ w257 w265 _]
              tunnel: w229 -> [_ w242 w250 _ _ _]
              frame #0 {
                n138 = Unbundle By Name(w233) -> ("move to origin button"=w234:bool)
                n139 = case shown="True" w234 {
                  tunnel: w235 -> [_ w236]
                  frame False {
                  }
                  frame True {
                    n140 = local read "Origin controls"() -> (w240:T3)
                    n141 = Unbundle By Name(w240) -> ("X"=w238:dbl, "Y"=w237:dbl)
                    n142 = call "IScanMoveXYZAbs.vi"("ZPos"=0.0, "YPos"=w237, "XPos"=w238, "PRIORLib.IScanIn"=w236) -> ()  [unwired: 3 out]
                  }
                }
              }
              frame #1 {
                n143 = Unbundle By Name(w244) -> ("Left"=w243:bool)
                n144 = case shown="True" w243 {
                  tunnel: w242 -> [_ w248]
                  tunnel: w241 -> [_ w245]
                  frame False {
                  }
                  frame True {
                    w246 = 0.0 ("ZPos")
                    n145 = Negate(x=w248) -> (-x=w247:i32)
                    n146 = call "IScanMoveXYZ.vi"("ZPos"=w246, "YPos"=w246, "XPos"=w247, "PRIORLib.IScanIn"=w245) -> ()  [unwired: 3 out]
                  }
                }
              }
              frame #2 {
                n147 = Unbundle By Name(w252) -> ("Right"=w251:bool)
                n148 = case shown="True" w251 {
                  tunnel: w250 -> [_ w254]
                  tunnel: w249 -> [_ w253]
                  frame False {
                  }
                  frame True {
                    w255 = 0.0 ("ZPos")
                    n149 = call "IScanMoveXYZ.vi"("ZPos"=w255, "YPos"=w255, "XPos"=w254, "PRIORLib.IScanIn"=w253) -> ()  [unwired: 3 out]
                  }
                }
              }
              frame #3 {
                n150 = Unbundle By Name(w259) -> ("Back"=w258:bool)
                n151 = case shown="True" w258 {
                  tunnel: w257 -> [_ w263]
                  tunnel: w256 -> [_ w260]
                  frame False {
                  }
                  frame True {
                    w261 = 0.0 ("ZPos")
                    n152 = Negate(x=w263) -> (-x=w262:i32)
                    n153 = call "IScanMoveXYZ.vi"("ZPos"=w261, "YPos"=w262, "XPos"=w261, "PRIORLib.IScanIn"=w260) -> ()  [unwired: 3 out]
                  }
                }
              }
              frame #4 {
                n154 = Unbundle By Name(w267) -> ("Forward"=w266:bool)
                n155 = case shown="True" w266 {
                  tunnel: w265 -> [_ w270]
                  tunnel: w264 -> [_ w268]
                  frame False {
                  }
                  frame True {
                    w269 = 0.0 ("ZPos")
                    n156 = call "IScanMoveXYZ.vi"("ZPos"=w269, "YPos"=w270, "XPos"=w269, "PRIORLib.IScanIn"=w268) -> ()  [unwired: 3 out]
                  }
                }
              }
              frame #5 {
                w272 = FALSE ("stage adjusted")
                # "restore all buttons"
                n157 = Bundle("stage adjusted"=w272, "stage adjusted"=w272, "stage adjusted"=w272, "stage adjusted"=w272, "stage adjusted"=w272) -> (w271:T18)  [unwired: 1 in]
                n158 = local write "Single step controls"(w271) -> ()
              }
            }
          }
        }
      }
      frame "Test init" {
        w298 = T17 0 items=["no dialog", "OK message", "continue or stop message", "OK message + warnings", "continue/stop + warnings"] ("type of dialog (OK msg:1)")
        # "Initialise scan map"
        # "Rescale histogram for 12-bit pixels"
        # "If an error occured, go straight to cleanup.\nOtherwise run the test."
        # "Stop camera if it's still running"
        # "Make controls inactive"
        # "check if file name is blank"
        n159 = local read "File name base"() -> (w313:string)
        n160 = Equal?(x=w313, y="<title>_<length>_<sampleID>_<stain>") -> (x = y?=w314:bool)
        n161 = case shown="True" w314 {
          tunnel: [errorcluster {"status"=FALSE, "code"=0, "source"=""} ("error out") w339] -> w310
          frame False {
          }
          frame True {
            n162 = call "No file name base given!"() -> ("File name base"=w340:string, "error out"=w339:errorcluster)  [unwired: 17 in, 1 out]
            n163 = local write "File name base"(w340) -> ()
          }
        }
        n164 = local read "camera button"() -> (w311:bool)
        n165 = case shown="True" w311 {
          tunnel: [errorcluster {"status"=FALSE, "code"=0, "source"=""} ("error out") w323] -> w304
          tunnel: w310 -> [_ w326]
          tunnel: w281 -> [_ w320]
          frame False {
          }
          frame True {
            n166 = Unbundle By Name(w320) -> ("Image Out"=w322:T7, "cameraID"=w325:u32)
            n167 = call <userlib>:"QCAM Grab Stop.vi"("error in (no error)"=w326, "cameraId"=w325) -> ("error out"=w327:errorcluster, "cameraId Out"=w328:u32)
            n168 = local write "camera button"(FALSE ("camera button")) -> ()
            n169 = call <userlib>:"QCAM Close.vi"("error in (no error)"=w327, "cameraId"=w328) -> ("error out"=w324:errorcluster)  [unwired: 1 in]
            n170 = call "IMAQ Dispose"("Image"=w322, "error in (no error)"=w324) -> ("error out"=w323:errorcluster)  [unwired: 4 in]
          }
        }
        n171 = stacked-sequence {
          tunnel: T10."Disabled and Grayed Out" ("Disabled") -> [w329 w330 w331 w332 w333 w334 w335 w336 w337]
          frame #0 {
            n172 = property on="Movement controls" class="Clust (strict)"("DisabledEnum"=w329) -> ()  [unwired: 2 in, 2 out]
          }
          frame #1 {
            n173 = property on="Preset controls" class="Clust (strict)"("DisabledEnum"=w330) -> ()  [unwired: 2 in, 2 out]
          }
          frame #2 {
            n174 = property on="Camera settings" class="Clust (strict)"("DisabledEnum"=w331) -> ()  [unwired: 2 in, 2 out]
          }
          frame #3 {
            n175 = property on="File name base" class="Str"("DisabledEnum"=w332) -> ()  [unwired: 2 in, 2 out]
          }
          frame #4 {
            n176 = property on="Image Output directory" class="Path"("DisabledEnum"=w333) -> ()  [unwired: 2 in, 2 out]
          }
          frame #5 {
            n177 = property on="Origin controls" class="Clust (strict)"("DisabledEnum"=w334) -> ()  [unwired: 2 in, 2 out]
          }
          frame #6 {
            n178 = property on="Single step controls" class="Clust (strict)"("DisabledEnum"=w335) -> ()  [unwired: 2 in, 2 out]
          }
          frame #7 {
            n179 = property on="camera button" class="Bool (strict)"("DisabledEnum"=w336) -> ()  [unwired: 2 in, 2 out]
          }
          frame #8 {
            n180 = property on="close button" class="Bool (strict)"("DisabledEnum"=w337) -> ()  [unwired: 2 in, 2 out]
          }
        }
        n181 = property on="Histogram" class="WFGraph (strict)"("XScale.Maximum"=4096.0 ("X Scale.Range:Maximum")) -> ()  [unwired: 2 in, 2 out]
        n182 = local read "File name base"() -> (w296:string)
        n183 = local read "Image Output directory"() -> (w301:path)
        n184 = Create Folder(path (use dialog)=w301) -> (created path=w300:path, error out=w299:errorcluster)  [unwired: 2 in, 1 out]
        n185 = Concatenate Strings(w296, "_focal_map.csv" ("name or relative path")) -> (w294:string)
        n186 = local read "Movement controls"() -> (w289:T2)
        n187 = call <vilib>:"Simple Error Handler.vi"("type of dialog (OK msg:1)"=w298, "error in (no error)"=w299) -> ()  [unwired: 3 in, 5 out]
        n188 = Build Path(base path=w300, name or relative path=w294) -> (appended path=w305:path)
        n189 = local read "No. of wells X"() -> (w286:i32)
        n190 = local read "No. of wells Y"() -> (w284:i32)
        n191 = Open/Create/Replace File(file path (use dialog)=w305, error in=w304, operation (0:open)=T13."replace or create", access (0:read/write)=enum16{"read/write", "read-only", "write-only"}."write-only") -> (refnum out=w302:refnum<file>, error out=w282:errorcluster)  [unwired: 2 in, 1 out]
        n192 = Unbundle By Name(w289) -> ("Nx"=w287:i32, "Ny"=w288:i32)
        n193 = Increment(x=w287) -> (x+1=w285:i32)
        n194 = Increment(x=w288) -> (x+1=w283:i32)
        n195 = Multiply(x=w286, y=w285) -> (x*y=w277:i32)
        n196 = Multiply(x=w284, y=w283) -> (x*y=w276:i32)
        n197 = Decrement(x=w277) -> (x-1=w274:i32)
        n198 = Decrement(x=w276) -> (x-1=w275:i32)
        n199 = Unbundle By Name(w281) -> ("Scan map"=w290:T7)
        n200 = call "IMAQ SetImageSize"("error in (no error)"=w282, "Y Resolution"=w275, "X Resolution"=w274, "Image"=w290) -> ("error out"=w291:errorcluster, "Image Out"=w293:T7)  [unwired: 1 in]
        n201 = call "IMAQ FillImage"("error in (no error)"=w291, "Pixel Value (U8, U16, I16, Float)"=i8 0, "Image"=w293) -> ("error out"=w279:errorcluster, "Image Out"=w273:T7)  [unwired: 7 in]
        n202 = local write "Scan map viewer"(w273) -> ()
        n203 = Bundle By Name(cluster=w281, "cameraID"=u32 0, "focal map fileref"=w302, "Scan map"=w273) -> (w280:T9)
        n204 = Tick Count (ms)() -> (millisecond timer value=w278:u32)
        n205 = local write "test start time"(w278) -> ()
        n206 = Unbundle By Name(w279) -> ("status"=w308:bool)
        n207 = Select(t=states_v2."Test clean", s=w308, f=states_v2."Test run") -> (s? t:f=w315:T8)
      }
      frame "Test run" {
        n208 = local read "No. of wells Y"() -> (w342:i32)
        n209 = for {
          N: w342 -> [_]
          tunnel: w341 -> [w345]
          i -> [w346]
          n210 = local read "No. of wells X"() -> (w347:i32)
          n211 = for {
            N: w347 -> [_]
            tunnel: w346 -> [w349]
            tunnel: w345 -> [w348]
            i -> [w350]
            n212 = local read "Movement controls"() -> (w352:T2)
            n213 = Unbundle By Name(w352) -> ("Ny"=w351:i32)
            n214 = for {
              N: w351 -> [_]
              tunnel: w350 -> [w355]
              tunnel: w349 -> [w354]
              tunnel: w348 -> [w353]
              i -> [w356]
              n215 = local read "Movement controls"() -> (w358:T2)
              n216 = Unbundle By Name(w358) -> ("Nx"=w357:i32)
              n217 = for {
                N: w357 -> [w359]
                tunnel: w356 -> [w365]
                tunnel: w355 -> [w362]
                tunnel: w354 -> [w363]
                tunnel: w353 -> [w361]
                i -> [w364]
                # "If test is aborted, go through the rest of the loop iterations, but do nothing"
                # "Wj"
                # "Wi"
                # "Nj"
                # "Ni"
                n218 = local read "abort test"() -> (w360:bool)
                n219 = case shown="False" w360 {
                  tunnel: w365 -> [w371 _]
                  tunnel: w364 -> [w370 _]
                  tunnel: w363 -> [w369 _]
                  tunnel: w362 -> [w368 _]
                  tunnel: w361 -> [w367 _]
                  tunnel: w359 -> [w366 _]
                  frame False {
                    # "true x index"
                    # "focus position, no. captures"
                    # "x,y"
                    n220 = stacked-sequence {
                      seq-local: [w379 _ _ _ _ _ _ _ _] -> [_ w407 _ _ _ _ _ _ w526]
                      seq-local: [_ _ _ w412 _ _ _ _ _] -> [_ _ _ _ _ _ _ w507 w517]
                      seq-local: [w372 _ _ _ _ _ _ _ _] -> [_ _ _ _ _ _ w492 _ w521]
                      tunnel: w371 -> [w376 _ _ _ _ w454 w500 _ w520]
                      tunnel: w370 -> [w374 _ _ _ _ w455 _ _ _]
                      tunnel: w369 -> [w393 _ _ _ _ w451 w501 _ w522]
                      tunnel: w368 -> [w392 _ _ _ _ w452 w499 _ w523]
                      tunnel: w367 -> [_ w410 _ w423 w436 w440 w495 w510 w514]
                      tunnel: w366 -> [w373 _ _ _ _ _ _ _ _]
                      frame #0 {
                        # "Change Ni on odd numbered\nrows, so the stage meanders"
                        # "calculate Y"
                        # "calculate X"
                        n221 = Quotient & Remainder(x=w376, y=2) -> (x-y*floor(x/y)=w377:i32)  [unwired: 1 out]
                        n222 = Equal To 0?(x=w377) -> (x = 0?=w375:bool)
                        n223 = case shown="False" w375 {
                          tunnel: w373 -> [w401 _]
                          tunnel: [w398 w402] -> w372
                          tunnel: w374 -> [w400 w402]
                          frame False {
                            n224 = Subtract(x=w401, y=w400) -> (x-y=w399:i32)
                            n225 = Decrement(x=w399) -> (x-1=w398:i32)
                          }
                          frame True {
                          }
                        }
                        n226 = local read "Movement controls"() -> (w397:T2)
                        n227 = local read "Well separation X"() -> (w391:dbl)
                        n228 = local read "Well separation Y"() -> (w394:dbl)
                        n229 = Unbundle By Name(w397) -> ("X separation"=w395:i32)
                        n230 = Unbundle By Name(w397) -> ("Y separation"=w396:i32)
                        n231 = local read "Origin controls"() -> (w386:T3)
                        n232 = Multiply(x=w391, y=w392) -> (x*y=w390:dbl)
                        n233 = Multiply(x=w395, y=w372) -> (x*y=w389:i32)
                        n234 = Multiply(x=w394, y=w393) -> (x*y=w387:dbl)
                        n235 = Multiply(x=w396, y=w376) -> (x*y=w388:i32)
                        n236 = Unbundle By Name(w386) -> ("X"=w384:dbl, "Y"=w382:dbl)
                        n237 = Add(x=w390, y=w389) -> (x+y=w383:dbl)
                        n238 = Add(x=w387, y=w388) -> (x+y=w385:dbl)
                        n239 = Add(x=w383, y=w384) -> (x+y=w381:dbl)
                        n240 = Add(x=w382, y=w385) -> (x+y=w380:dbl)
                        n241 = Bundle(w381, w380) -> (w379:cluster{dbl, dbl})  [unwired: 1 in]
                      }
                      frame #1 {
                        # "move"
                        n242 = Unbundle By Name(w410) -> ("PRIORLib.IScanOut"=w409:refnum<k7>)
                        n243 = Unbundle(w407) -> (w406:dbl, w405:dbl)
                        n244 = call "IScanMoveXYZAbs.vi"("ZPos"=0.0, "YPos"=w405, "XPos"=w406, "PRIORLib.IScanIn"=w409) -> ("error out"=w403:errorcluster, "PRIORLib.IScanOut"=w404:refnum<k7>)  [unwired: 1 out]
                        n245 = call "wait_for_movement.vi"("error in (no error)"=w403, "IScan in"=w404) -> ()  [unwired: 9 in, 1 out]
                      }
                      frame #2 {
                        # "Extra wait fro CCD to settle"
                        n246 = local read "Additional delay between captures (ms)"() -> (w411:dbl)
                        n247 = Wait (ms)(milliseconds to wait=w411) -> ()  [unwired: 1 out]
                      }
                      frame #3 {
                        # "open camera for focusing"
                        # "Reset camera ID"
                        # "Close camera"
                        # "autofocus"
                        n248 = local read "Camera settings"() -> (w424:T5)
                        n249 = call "start_camera_new.vi"("image type"=image_type."preview_image", "Camera settings"=w424) -> ("cameraId out"=w426:u32, "Refnum out"=w427:T7)  [unwired: 6 in, 2 out]
                        n250 = Bundle By Name(cluster=w423, "Image Out"=w427, "cameraID"=w426) -> (w422:T9)
                        n251 = call "autofocus.vi"("dynamic scope variables"=w422) -> ("dynamic scope variables out"=w417:T9, "Focus position"=w414:dbl, "Number of captures"=w413:i32)  [unwired: 1 in]
                        n252 = Bundle("Focus position"=w414, "Number of captures"=w413) -> (w412:T19)  [unwired: 1 in]
                        n253 = Unbundle By Name(w417) -> ("Image Out"=w419:T7, "cameraID"=w420:u32)
                        n254 = call <userlib>:"QCAM Grab Stop.vi"("cameraId"=w420) -> ("error out"=w415:errorcluster, "cameraId Out"=w421:u32)  [unwired: 1 in]
                        n255 = call <userlib>:"QCAM Close.vi"("error in (no error)"=w415, "cameraId"=w421) -> ("error out"=w416:errorcluster)  [unwired: 1 in]
                        n256 = call "IMAQ Dispose"("Image"=w419, "error in (no error)"=w416) -> ()  [unwired: 4 in, 1 out]
                        n257 = Bundle By Name(cluster=w417, "cameraID"=u32 0) -> ()  [unwired: 1 out]
                      }
                      frame #4 {
                        # "go to most downward stack position"
                        n258 = Unbundle By Name(w436) -> ("PRIORLib.IScanOut"=w429:refnum<k7>, "PRIORLib.IZOut"=w430:refnum<k7>)
                        n259 = local read "No. of images in focal stack"() -> (w435:i32)
                        n260 = local read "Focal stack separation"() -> (w432:dbl)
                        n261 = Quotient & Remainder(x=w435, y=2) -> (floor(x/y)=w433:i32)  [unwired: 1 out]
                        n262 = Multiply(x=w433, y=w432) -> (x*y=w431:dbl)
                        n263 = call "IZMoveDown.vi"("Distance"=w431, "PRIORLib.IZIn"=w430) -> ("error out"=w428:errorcluster)  [unwired: 1 in, 2 out]
                        n264 = call "wait_for_movement.vi"("error in (no error)"=w428, "IScan in"=w429) -> ()  [unwired: 9 in, 1 out]
                      }
                      frame #5 {
                        # "Capture all images in focal stack"
                        n265 = local read "No. of images in focal stack"() -> (w453:i32)
                        n266 = local read "Camera settings"() -> (w449:T5)
                        n267 = local read "Well numbering mode"() -> (w444:u16)
                        n268 = call "start_camera_new.vi"("image type"=image_type."capture_image", "Camera settings"=w449) -> ("cameraId out"=w443:u32, "Refnum out"=w442:T7)  [unwired: 6 in, 2 out]
                        n269 = Unbundle By Name(w440) -> ("PRIORLib.IScanOut"=w439:refnum<k7>, "PRIORLib.IZOut"=w438:refnum<k7>)
                        n270 = for {
                          N: w453 -> [_]
                          tunnel: w455 -> [w471]
                          tunnel: w454 -> [w472]
                          tunnel: w452 -> [w476]
                          tunnel: w451 -> [w475]
                          tunnel: [w462] -> w445
                          tunnel: w444 -> [w474]
                          tunnel: w443 -> [w467]
                          tunnel: [w456] -> w441
                          tunnel: w439 -> [w458]
                          tunnel: w438 -> [w463]
                          shift-right: [w461] -> w437
                          shift-left: w442 -> [w466]
                          i -> [w473]
                          # "Handle numbering mode"
                          n271 = case shown="1, Default" w474 {
                            tunnel: w476 -> [w483 w491]
                            tunnel: w475 -> [w482 w487]
                            tunnel: [w481 w489] -> w477
                            frame 0 {
                              n272 = call "Build Text2"("Beginning Text"="", "Wi"=w483, "Wj"=w482) -> ("Result"=w481:string)  [unwired: 11 in, 1 out]
                            }
                            frame 1, Default {
                              # "make well letter\nfrom number"
                              n273 = Add(x=65, y=w491) -> (x+y=w486:i32)
                              n274 = To Byte Integer(number=w486) -> (8bit integer=w485:i8)
                              n275 = Type Cast(x=w485) -> (*(type *) &x=w488:string)  [unwired: 1 in]
                              n276 = call "Build Text"("Beginning Text"=w488, "well_j"=w487) -> ("Result"=w489:string)  [unwired: 12 in, 1 out]
                            }
                          }
                          n277 = local read "File name base"() -> (w479:string)
                          n278 = local read "Image Output directory"() -> (w470:path)
                          n279 = call "Build Text"("Beginning Text"=w479, "Nk"=w473, "cell"=w477, "Ni"=w471, "Nj"=w472) -> ("Result"=w478:string, "error out"=w469:errorcluster)  [unwired: 9 in]
                          n280 = Build Path(base path=w470, name or relative path=w478) -> (appended path=w468:path)
                          n281 = call <userlib>:"QCAM Grab Acquire.vi"("error in (no error)"=w469, "Image"=w466, "cameraId"=w467) -> ("error out"=w459:errorcluster, "Image Out"=w460:T7, "cameraId out"=w462:u32)
                          n282 = call-poly "IMAQ Write File 2"("error in (no error)"=w459, "File Path"=w468, "Image"=w460) -> ("error out"=w464:errorcluster, "Image Out (duplicate)"=w461:T7)  [unwired: 7 in]
                          n283 = local read "Focal stack separation"() -> (w465:dbl)
                          n284 = call "IMAQ Histograph"("Image"=w461) -> ("Histogram Graph"=w480:T6)  [unwired: 7 in, 3 out]
                          n285 = local write "Preview"(w461) -> ()
                          n286 = local write "Histogram"(w480) -> ()
                          n287 = call "IZMoveUp.vi"("Distance"=w465, "error in (no error)"=w464, "PRIORLib.IZIn"=w463) -> ("error out"=w457:errorcluster)  [unwired: 2 out]
                          n288 = call "wait_for_movement.vi"("error in (no error)"=w457, "IScan in"=w458) -> ("error out"=w456:errorcluster)  [unwired: 9 in]
                        }
                        n289 = call <userlib>:"QCAM Grab Stop.vi"("error in (no error)"=w441, "cameraId"=w445) -> ("error out"=w447:errorcluster, "cameraId Out"=w448:u32)
                        n290 = call <userlib>:"QCAM Close.vi"("error in (no error)"=w447, "cameraId"=w448) -> ("error out"=w446:errorcluster)  [unwired: 1 in]
                        n291 = call "IMAQ Dispose"("Image"=w437, "error in (no error)"=w446) -> ()  [unwired: 4 in, 1 out]
                      }
                      frame #6 {
                        # "Set pixel on scan map"
                        n292 = local read "Movement controls"() -> (w498:T2)
                        n293 = Unbundle By Name(w498) -> ("Nx"=w497:i32, "Ny"=w496:i32)
                        n294 = Unbundle By Name(w495) -> ("Scan map"=w494:T7)
                        n295 = formula code="int32 x;\nint32 y;\n\nx = (Wi*(nx+1)) +ni;\ny = (Wj*(ny+1)) +nj;"("nx"=w497, "ny"=w496, "Wi"=w499, "Wj"=w501, "ni"=w492, "nj"=w500) -> ("x"=w503:i32, "y"=w504:i32)
                        n296 = call "IMAQ SetPixelValue"("Pixel Value"=u8 255, "Y Coordinate"=w504, "X Coordinate"=w503, "Image"=w494) -> ("Image Out"=w493:T7)  [unwired: 6 in, 1 out]
                        n297 = local write "Scan map viewer"(w493) -> ()
                      }
                      frame #7 {
                        # "Handle case that no cells are present"
                        # "return to original focus position"
                        n298 = Unbundle By Name(w510) -> ("PRIORLib.IScanOut"=w508:refnum<k7>, "PRIORLib.IZOut"=w509:refnum<k7>)
                        n299 = Unbundle(w507) -> ("Focus position"=w506:dbl)  [unwired: 1 out]
                        n300 = Not A Number/Path/Refnum?(number/path/refnum=w506) -> (NaN/Path/Refnum?=w505:bool)
                        n301 = case shown="False" w505 {
                          tunnel: w509 -> [w513 _]
                          tunnel: w508 -> [w512 _]
                          frame False {
                            n302 = call "IZMoveAbs.vi"("PRIORLib.IZIn"=w513) -> ("error out"=w511:errorcluster)  [unwired: 1 in, 2 out]
                            n303 = call "wait_for_movement.vi"("error in (no error)"=w511, "IScan in"=w512) -> ()  [unwired: 9 in, 1 out]
                          }
                          frame True {
                          }
                        }
                      }
                      frame #8 {
                        # "Wi, Wj, Ni, Nj, absX, absY, Z, no. of captures"
                        # "Save focus postion to focal map file"
                        # "check exit conditions"
                        n304 = Unbundle By Name(w514) -> ("focal map fileref"=w525:refnum<file>)
                        n305 = local read "Run test button"() -> (w528:bool)
                        n306 = global read "Globals.vi" "EmerStop"() -> (w530:bool)
                        n307 = Unbundle(w526) -> (w519:dbl, w518:dbl)
                        n308 = Unbundle(w517) -> ("Focus position"=w516:dbl, "Number of captures"=w515:i32)
                        n309 = Not(x=w528) -> (.not. x?=w527:bool)
                        n310 = Format Into String(format string="%d,%d,%d,%d,%f,%f,%f,%d\\n", initial string=w525, w523, w522, w521, w520, w519, w518, w516, w515) -> ()  [unwired: 1 in, 2 out]
                        n311 = Compound Arithmetic op=OR(w527, w530) -> (→"abort test":bool)
                      }
                    }
                  }
                  frame True {
                  }
                }
              }
            }
          }
        }
      }
      frame "Test clean" {
        w540 = FALSE ("Run test button")
        # "Close focal map file"
        # "Return to origin"
        # "Rescale histogram for 8-bit pixels"
        # "Reset camera ID"
        # "Reset button"
        # "Make controls active again"
        n312 = stacked-sequence {
          tunnel: T10."Enabled" ("Disabled") -> [w547 w548 w549 w550 w551 w552 w553 w554 w555]
          frame #0 {
            n313 = property on="Movement controls" class="Clust (strict)"("DisabledEnum"=w547) -> ()  [unwired: 2 in, 2 out]
          }
          frame #1 {
            n314 = property on="Preset controls" class="Clust (strict)"("DisabledEnum"=w548) -> ()  [unwired: 2 in, 2 out]
          }
          frame #2 {
            n315 = property on="Camera settings" class="Clust (strict)"("DisabledEnum"=w549) -> ()  [unwired: 2 in, 2 out]
          }
          frame #3 {
            n316 = property on="File name base" class="Str"("DisabledEnum"=w550) -> ()  [unwired: 2 in, 2 out]
          }
          frame #4 {
            n317 = property on="Image Output directory" class="Path"("DisabledEnum"=w551) -> ()  [unwired: 2 in, 2 out]
          }
          frame #5 {
            n318 = property on="Origin controls" class="Clust (strict)"("DisabledEnum"=w552) -> ()  [unwired: 2 in, 2 out]
          }
          frame #6 {
            n319 = property on="Single step controls" class="Clust (strict)"("DisabledEnum"=w553) -> ()  [unwired: 2 in, 2 out]
          }
          frame #7 {
            n320 = property on="camera button" class="Bool (strict)"("DisabledEnum"=w554) -> ()  [unwired: 2 in, 2 out]
          }
          frame #8 {
            n321 = property on="close button" class="Bool (strict)"("DisabledEnum"=w555) -> ()  [unwired: 2 in, 2 out]
          }
        }
        n322 = local read "Origin controls"() -> (w538:T3)
        n323 = Unbundle By Name(w534) -> ("focal map fileref"=w533:refnum<file>)
        n324 = Unbundle By Name(w534) -> ("PRIORLib.IScanOut"=w535:refnum<k7>)
        n325 = Unbundle By Name(w538) -> ("X"=w537:dbl, "Y"=w536:dbl)
        n326 = Close File(refnum=w533) -> ()  [unwired: 1 in, 2 out]
        n327 = local write "Run test button"(w540) -> ()
        n328 = local write "abort test"(w540) -> ()
        n329 = call "IScanMoveXYZAbs.vi"("ZPos"=0.0, "YPos"=w536, "XPos"=w537, "PRIORLib.IScanIn"=w535) -> ("error out"=w532:errorcluster)  [unwired: 2 out]
        n330 = Bundle By Name(cluster=w534, "cameraID"=u32 0) -> (w542:T9)
        n331 = call "Display Message to User"("error in (no error)"=w532) -> ("error out"=w531:errorcluster)  [unwired: 9 in, 1 out]
        n332 = property on="Histogram" class="WFGraph (strict)"("XScale.Maximum"=255.0 ("X Scale.Range:Maximum")) -> ()  [unwired: 2 in, 2 out]
      }
      frame "Close" {
        # "Close camera connection"
        # "Turn off connection indicator"
        # "Set buttons to off"
        # "Close connections to stage"
        n333 = Unbundle By Name(w558) -> ("PRIORLib.IScanOut"=w561:refnum<k7>, "PRIORLib.IStageOut"=w562:refnum<k7>, "PRIORLib.IFilterOut"=w564:refnum<k7>, "PRIORLib.IZOut"=w563:refnum<k7>)
        n334 = stacked-sequence {
          tunnel: w558 -> [_ w572]
          tunnel: [_ w568] -> w556
          frame #0 {
            n335 = global write "QCam Grab Abort.vi" "Grab Abort"(TRUE ("Grab Abort")) -> ()
          }
          frame #1 {
            n336 = Unbundle By Name(w572) -> ("cameraID"=w570:u32, "Image Out"=w569:T7)
            n337 = Not Equal To 0?(x=w570) -> (x != 0?=w571:bool)
            n338 = case shown="False" w571 {
              tunnel: w570 -> [_ w576]
              tunnel: w569 -> [_ w575]
              tunnel: [_ w573] -> w568
              frame False {
              }
              frame True {
                n339 = call <userlib>:"QCAM Grab Stop.vi"("cameraId"=w576) -> ("error out"=w577:errorcluster, "cameraId Out"=w578:u32)  [unwired: 1 in]
                n340 = call <userlib>:"QCAM Close.vi"("error in (no error)"=w577, "cameraId"=w578) -> ("error out"=w574:errorcluster)  [unwired: 1 in]
                n341 = call "IMAQ Dispose"("Image"=w575, "error in (no error)"=w574) -> ("error out"=w573:errorcluster)  [unwired: 4 in]
              }
            }
          }
        }
        n342 = stacked-sequence {
          tunnel: w561 -> [_ _ _ w590]
          tunnel: w562 -> [_ _ w589 _]
          tunnel: w564 -> [w587 _ _ _]
          tunnel: w563 -> [_ w588 _ _]
          frame #0 {
            n343 = call "IFilterClose.vi"("PRIORLib.IFilter"=w587) -> ()  [unwired: 1 out]
          }
          frame #1 {
            n344 = call "IZClose.vi"("PRIORLib.IZ"=w588) -> ()  [unwired: 1 out]
          }
          frame #2 {
            n345 = call "IStageClose.vi"("PRIORLib.IStage"=w589) -> ()  [unwired: 1 out]
          }
          frame #3 {
            n346 = call "IScanClose.vi"("PRIORLib.IScan"=w590) -> ()  [unwired: 2 out]
          }
        }
        n347 = stacked-sequence {
          tunnel: FALSE ("Value") -> [w579 w580 w581 w582 w583 w584 w585]
          frame #0 {
            n348 = property on="auto expose button" class="Bool (strict)"("Value"=w579) -> ()  [unwired: 2 in, 2 out]
          }
          frame #1 {
            n349 = property on="set origin button" class="Bool (strict)"("Value"=w580) -> ()  [unwired: 2 in, 2 out]
          }
          frame #2 {
            n350 = property on="save preset button" class="Bool (strict)"("Value"=w581) -> ()  [unwired: 2 in, 2 out]
          }
          frame #3 {
            n351 = property on="Run test button" class="Bool (strict)"("Value"=w582) -> ()  [unwired: 2 in, 2 out]
          }
          frame #4 {
            n352 = property on="close button" class="Bool (strict)"("Value"=w583) -> ()  [unwired: 2 in, 2 out]
          }
          frame #5 {
            n353 = property on="camera button" class="Bool (strict)"("Value"=w584) -> ()  [unwired: 2 in, 2 out]
          }
          frame #6 {
            n354 = Bundle("Value"=w585, "Value"=w585, "Value"=w585, "Value"=w585, "Value"=w585) -> (w586:T15)  [unwired: 1 in]
            n355 = property on="Single step controls" class="Clust (strict)"("Value"=w586) -> ()  [unwired: 2 in, 2 out]
          }
        }
        n356 = local write "connection indicator"(FALSE ("connection indicator")) -> ()
      }
    }
    "error display" <- w3
    n357 = Wait (ms)(milliseconds to wait=u32 50) -> ()  [unwired: 1 out]
  }
  n358 = while {
    i -> [w591]
    stop <- w593 stop-if-true
    n359 = event shown="[0] Timeout" {
      selector: _ -> [_ _ _]
      dyn-events: _ -> [_ _ _]
      timeout: 25 -> [_ _ _]
      tunnel: w591 -> [w599 _ _]
      event Timeout {
        # "Displsy time if on emergency stop"
        n360 = event-data() -> ()  [unwired: 1 in, 2 out]
        n361 = local read "Run test button"() -> (w595:bool)
        n362 = Quotient & Remainder(x=w599, y=40) -> (x-y*floor(x/y)=w597:i32)  [unwired: 1 out]
        n363 = Equal To 0?(x=w597) -> (x = 0?=w596:bool)
        n364 = And(x=w595, y=w596) -> (x .and. y?=w594:bool)
        n365 = case shown="True" w594 {
          frame False {
          }
          frame True {
            n366 = local read "Scan map viewer"() -> (w600:T7)
            n367 = Tick Count (ms)() -> (millisecond timer value=w604:u32)
            n368 = call "time_display.vi"("scan map in"=w600, "test start time"="test start time", "millisecond timer value"=w604) -> ("estimated time remaining"=→"estimated remaining":string, "elapsed time"=→"elapsed time":string)  [unwired: 7 in]
          }
        }
      }
      event Key Down {
        n369 = event-data() -> ("VKey"=w607:T20)  [unwired: 1 in, 5 out]
        n370 = Equal?(x=eventvkey."Escape", y=w607) -> (x = y?=w605:bool)
        n371 = case shown="True" w605 {
          frame False {
          }
          frame True {
            n372 = call "Display Message to User3"() -> ()  [unwired: 10 in, 2 out]
            n373 = global write "Globals.vi" "EmerStop"(TRUE) -> ()
          }
        }
      }
      event "emergency stop": Value Change {
        n374 = event-data() -> ("NewVal"=w609:bool)  [unwired: 1 in, 4 out]
        n375 = case shown="True" w609 {
          frame False {
          }
          frame True {
            n376 = call "Display Message to User2"() -> ()  [unwired: 10 in, 2 out]
            n377 = global write "Globals.vi" "EmerStop"(TRUE) -> ()
          }
        }
      }
    }
    n378 = local read "close button"() -> (w593:bool)
  }
